vi "SunplusDailyYY.vi"() -> ()   [LabVIEW 2012]
uses:
  <vilib>/addons/database/Auxilliary.llb/DB Tools Cursor Type.ctl
  <vilib>/Utility/NIReport.llb/NI_report.lvclass
  <vilib>/addons/database/Connection.llb/DB Tools Open Connec (Path).vi
  <vilib>/addons/database/Connection.llb/Conn Execute.vi
  <vilib>/addons/database/Recordset.llb/Rec Fetch Recordset Data (R).vi
  <vilib>/addons/database/Recordset.llb/Rec Destroy - Connection.vi
  <vilib>/addons/database/_DB Variant To Data/Database Variant To Data.xnode
  <vilib>/addons/database/NI_Database_API.lvlib
  <vilib>/Utility/NIReport.llb/Excel/NI_Excel.lvclass
  <vilib>/Utility/SMTP/NI_SMTPEmail.lvlib
panel:
  out "error out 2":errorcluster
  in  "MIME content-type (application/octet-stream)":string="application/octet-stream"
  out "error out 4":errorcluster
  in  "?":cluster{"start row":i32, "start column":i32}
  out "error out":errorcluster
  in  "start (0, 0)":cluster{"start row":i32, "start column":i32}
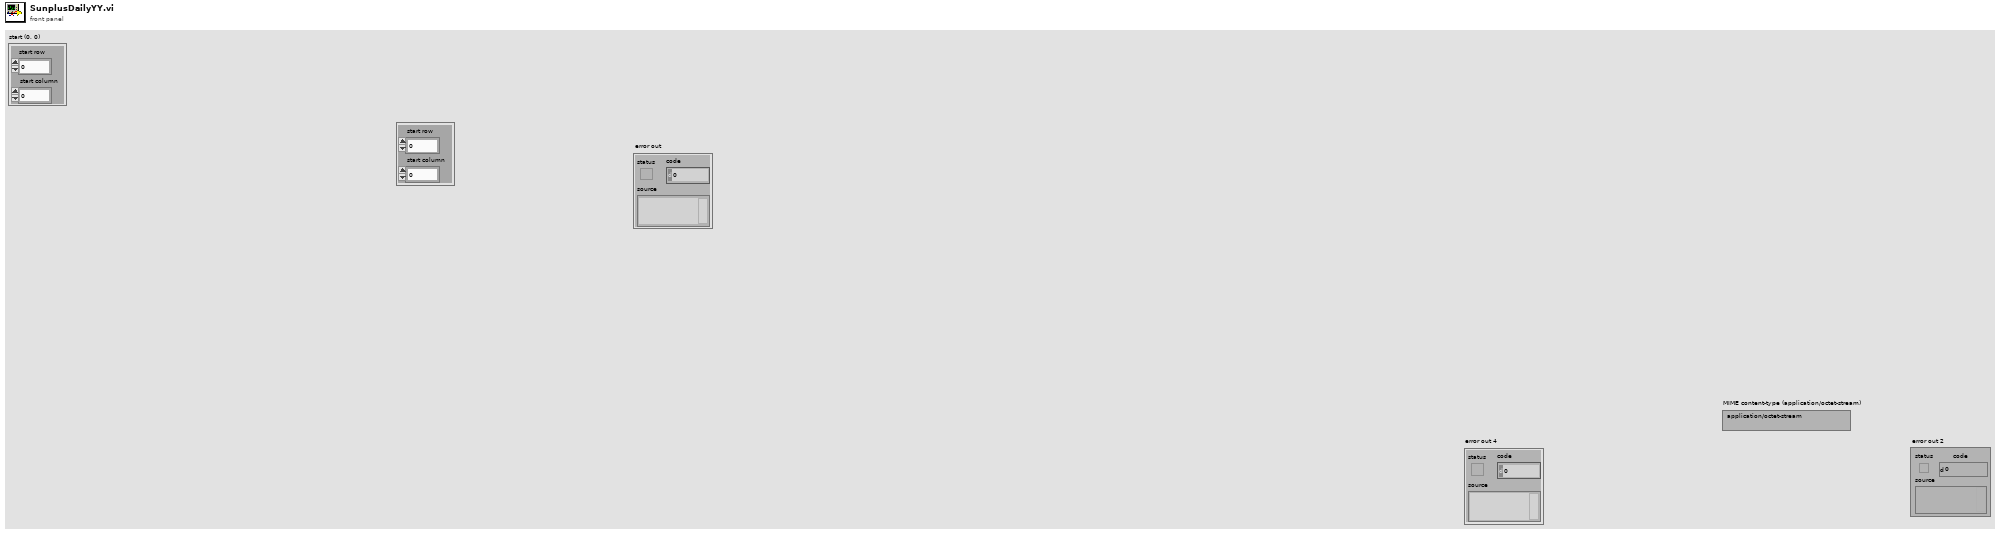
[diagram p1: front panel]
types:
  T1 = typedef "NI_Database_API.lvlib/DB Tools Cursor Type.ctl" = enum16{"forward-only", "keyset", "dynamic", "static"}
  T2 = enum16{"Standard Report", "HTML", "Word", "Excel"}
  T3 = typedef "NI_Database_API.lvlib/Conn ObjectReference.ctl" = refnum<k1>
  T4 = typedef "NI_Database_API.lvlib/Rec ObjectReference.ctl" = refnum<k1>
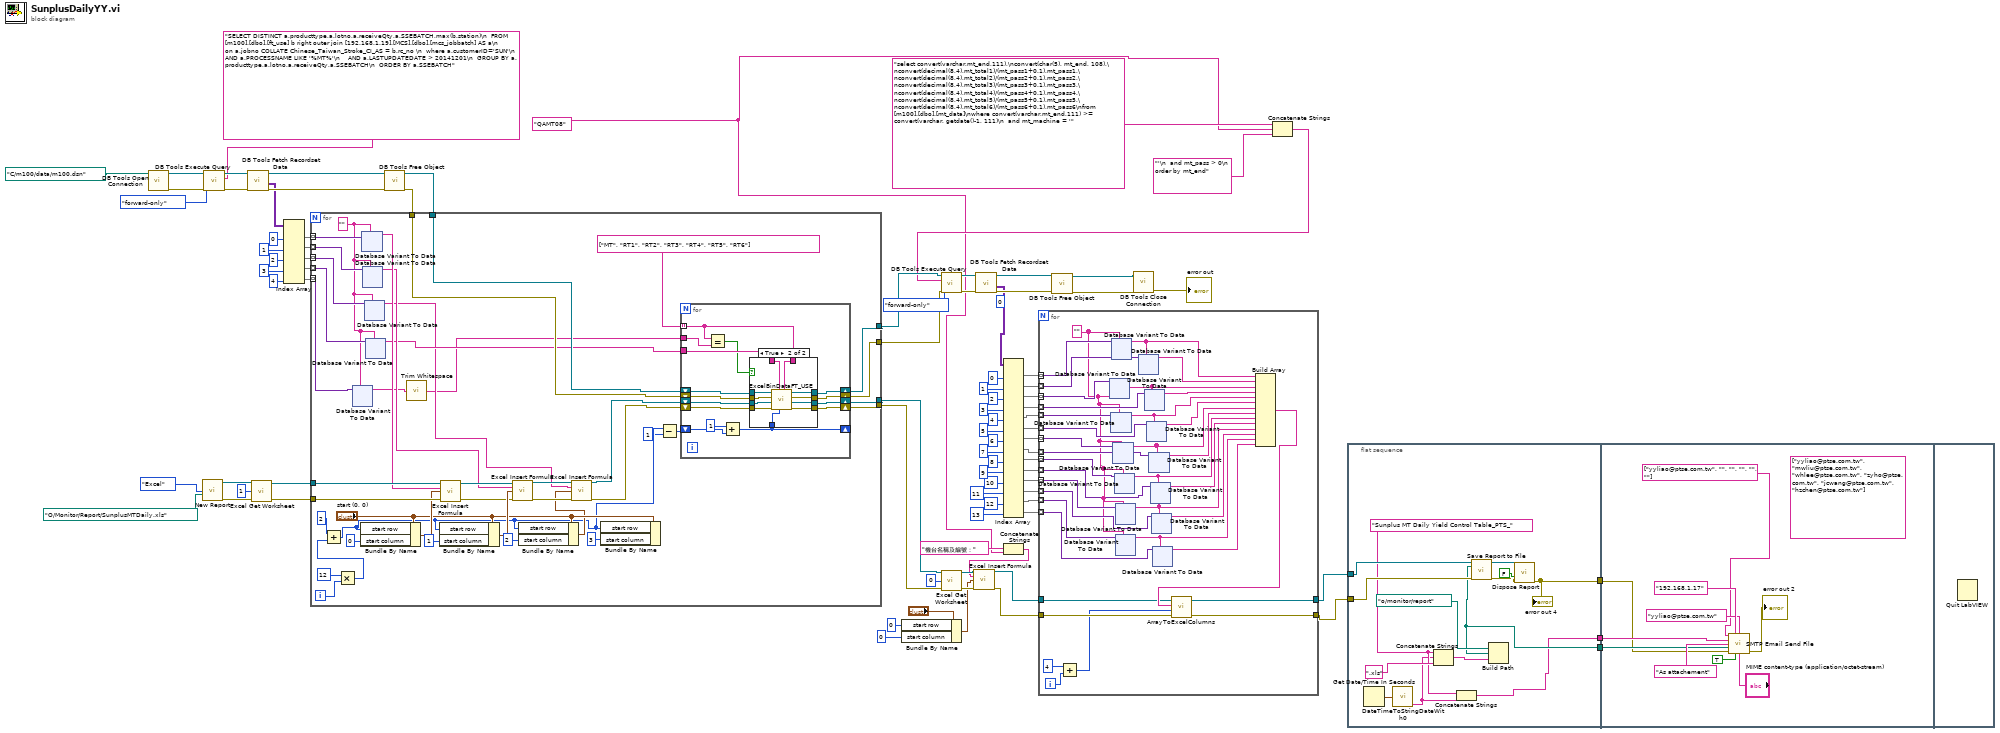
[diagram p0: block diagram]
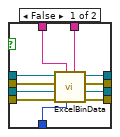
[diagram p2: hidden frame]
diagram:
  w6 = "QAMT08" ("Machine")
  (unwired) 0 ("index")
  n1 = call-poly <vilib>:"DB Tools Open Connection.vi"("connection information"=path "C:/m100/data/m100.dsn") -> ("error out"=w82:errorcluster, "connection reference"=w83:T3)  [unwired: 7 in]
  n2 = call <vilib>:"New Report.vi"("report type"=T2."Excel" ("Report Type"), "template (empty)"=path "O:/Monitor/Report/SunplusMTDaily.xls") -> ("report out"=w67:refnum<class "NI_report.lvclass">, "error out"=w66:errorcluster)  [unwired: 12 in]
  n3 = call-poly <vilib>:"DB Tools Execute Query.vi"("error in (no error)"=w82, "cursor type"=DB_Tools_Cursor_Type."forward-only", "SQL query"="SELECT DISTINCT a.producttype,a.lotno,a.receiveQty,a.SSEBATCH,max(b.station)\n  FROM [m100].[dbo].[ft_use] b right outer join [192.168.1.19].[MCS].[dbo].[mcs_jobbatch] AS a\n  on a.jobno COLLATE Chinese_Taiwan_Stroke_CI_AS = b.rc_no \n  where a.customerID='SUN'\n    AND a.PROCESSNAME LIKE '%MT%'\n    AND a.LASTUPDATEDATE > 20141201\n  GROUP BY a.producttype,a.lotno,a.receiveQty,a.SSEBATCH\n  ORDER BY a.SSEBATCH", "connection reference"=w83) -> ("error out"=w84:errorcluster, "recordset reference"=w85:T4)  [unwired: 4 in]
  n4 = call-poly <vilib>:"DB Tools Fetch Recordset Data.vi"("error in (no error)"=w84, "recordset reference"=w85) -> ("error out"=w86:errorcluster, "recordset data"=w79:variant[][], "recordset reference out"=w87:T4)  [unwired: 3 in]
  n5 = call <vilib>:"Excel Get Worksheet.vi"("report in"=w67, "worksheet index (0)"=1, "error in (no error)"=w66) -> ("report out"=w63:refnum<class "NI_report.lvclass">, "error out"=w62:errorcluster)  [unwired: 11 in]
  n6 = Index Array(array=w79, index (col) #1=0 ("disabled index (col)"), index (col) #2=1 ("index (col)"), index (col) #3=2 ("index (col)"), index (col) #4=3 ("index (col)"), index (col) #5=4 ("index (col)")) -> (element #1=w75:variant[], element #2=w74:variant[], element #3=w73:variant[], element #4=w69:variant[], element #5=w1:variant[])  [unwired: 5 in]
  n7 = call-poly <vilib>:"DB Tools Free Object.vi"("error in (no error)"=w86, "recordset reference"=w87) -> ("error out"=w72:errorcluster, "connection reference"=w71:T3)  [unwired: 8 in]
  n8 = for {
    tunnel: w75 -> [w132] mode=indexing
    tunnel: w74 -> [w131] mode=indexing
    tunnel: w73 -> [w130] mode=indexing
    tunnel: w72 -> [w107]
    tunnel: w71 -> [w108]
    tunnel: w69 -> [w129] mode=indexing
    tunnel: w63 -> [w128]
    tunnel: w62 -> [w127]
    tunnel: [w98] -> w61
    tunnel: [w97] -> w60
    tunnel: [w100] -> w52
    tunnel: [w99] -> w51
    tunnel: w1 -> [w94] mode=indexing
    i -> [w111]
    w93 = ""
    n9 = Multiply(x=12, y=w111) -> (x*y=w109:i32)
    n10 = Add(x=2, y=w109) -> (x+y=w104:i32)
    n11 = xnode "Database Variant To Data"("database variant"=w94, "type"=w93) -> ("data"=w92:string)  [unwired: 1 in, 1 out]
    n12 = Bundle By Name(cluster="start (0, 0)", "start row"=w104, "start column"=0) -> (w126:cluster{"start row":i32, "start column":i32})
    n13 = xnode "Database Variant To Data"("database variant"=w132, "type"=w93) -> ("data"=w123:string)  [unwired: 1 in, 1 out]
    n14 = xnode "Database Variant To Data"("database variant"=w131, "type"=w93) -> ("data"=w118:string)  [unwired: 1 in, 1 out]
    n15 = xnode "Database Variant To Data"("database variant"=w130, "type"=w93) -> ("data"=w95:string)  [unwired: 1 in, 1 out]
    n16 = xnode "Database Variant To Data"("database variant"=w129, "type"=w93) -> ("data"=w101:string)  [unwired: 1 in, 1 out]
    n17 = call <vilib>:"Trim Whitespace.vi"("string"=w92) -> ("trimmed string"=w91:string)  [unwired: 1 in]
    n18 = Bundle By Name(cluster="start (0, 0)", "start row"=w104, "start column"=1) -> (w121:cluster{"start row":i32, "start column":i32})
    n19 = call <vilib>:"Excel Insert Formula.vi"("report in"=w128, "formula"=w123, "start (0, 0)"=w126, "error in (no error)"=w127) -> ("report out"=w120:refnum<class "NI_report.lvclass">, "error out"=w119:errorcluster)  [unwired: 10 in]
    n20 = call <vilib>:"Excel Insert Formula.vi"("report in"=w120, "formula"=w118, "start (0, 0)"=w121, "error in (no error)"=w119) -> ("report out"=w116:refnum<class "NI_report.lvclass">, "error out"=w115:errorcluster)  [unwired: 10 in]
    n21 = Bundle By Name(cluster="start (0, 0)", "start row"=w104, "start column"=2) -> (w112:cluster{"start row":i32, "start column":i32})
    n22 = call <vilib>:"Excel Insert Formula.vi"("report in"=w116, "formula"=w95, "start (0, 0)"=w112, "error in (no error)"=w115) -> ("report out"=w106:refnum<class "NI_report.lvclass">, "error out"=w105:errorcluster)  [unwired: 10 in]
    n23 = Bundle By Name(cluster="start (0, 0)", "start row"=w104, "start column"=3) -> ()  [unwired: 1 out]
    n24 = Subtract(x=w104, y=1) -> (x-y=w102:i32)
    n25 = for {
      shift-right: [w178] -> w100
      shift-left: w108 -> [w171]
      shift-right: [w177] -> w99
      shift-left: w107 -> [w170]
      shift-right: [w176] -> w98
      shift-left: w106 -> [w169]
      shift-right: [w175] -> w97
      shift-left: w105 -> [w168]
      shift-right: [w174] -> _
      shift-left: w102 -> [w173]
      tunnel: w101 -> [w172]
      tunnel: string[] ["MT", "RT1", "RT2", "RT3", "RT4", "RT5", "RT6"] ("Array") -> [w166] mode=indexing
      tunnel: w91 -> [w167]
      n26 = Equal?(x=w166, y=w167) -> (x = y?=w165:bool)
      n27 = Add(x=1, y=w173) -> (x+y=w174:i32)
      n28 = case shown="True" w165 {
        tunnel: [w190 w196] -> w178
        tunnel: [w189 w195] -> w177
        tunnel: [w188 w194] -> w176
        tunnel: [w187 w193] -> w175
        tunnel: w174 -> [w186 w201]
        tunnel: w172 -> [w185 w192]
        tunnel: w171 -> [w184 w200]
        tunnel: w170 -> [w183 w199]
        tunnel: w169 -> [w182 w198]
        tunnel: w168 -> [w181 w197]
        tunnel: w166 -> [w180 w191]
        frame False {
          n29 = call "ExcelBinData.vi"("step"=w180, "start row"=w186, "jobno"=w185, "error in (no error) 2"=w181, "report in"=w182, "error in (no error)"=w183, "connection reference 2"=w184) -> ("error out 2"=w187:errorcluster, "report out"=w188:refnum<class "NI_report.lvclass">, "error out"=w189:errorcluster, "connection reference"=w190:T3)  [unwired: 1 in]
        }
        frame True {
          n30 = call "ExcelBinDataFT_USE.vi"("step"=w191, "start row"=w201, "jobno"=w192, "error in (no error) 2"=w197, "report in"=w198, "error in (no error)"=w199, "connection reference 2"=w200) -> ("error out 2"=w193:errorcluster, "report out"=w194:refnum<class "NI_report.lvclass">, "error out"=w195:errorcluster, "connection reference"=w196:T3)  [unwired: 1 in]
        }
      }
    }
  }
  n31 = Bundle By Name(cluster="?", "start row"=0, "start column"=0) -> (w11:cluster{"start row":i32, "start column":i32})
  n32 = call <vilib>:"Excel Get Worksheet.vi"("report in"=w61, "worksheet index (0)"=0, "error in (no error)"=w60) -> ("report out"=w16:refnum<class "NI_report.lvclass">, "error out"=w15:errorcluster)  [unwired: 11 in]
  n33 = Concatenate Strings("機台名稱及編號：" ("formula"), w6) -> (w8:string)
  n34 = call <vilib>:"Excel Insert Formula.vi"("report in"=w16, "formula"=w8, "start (0, 0)"=w11, "error in (no error)"=w15) -> ("report out"=w10:refnum<class "NI_report.lvclass">, "error out"=w9:errorcluster)  [unwired: 10 in]
  n35 = Concatenate Strings("select convert(varchar,mt_end,111),\nconvert(char(5), mt_end, 108),\nconvert(decimal(8,4),mt_total1)/(mt_pass1+0.1),mt_pass1,\nconvert(decimal(8,4),mt_total2)/(mt_pass2+0.1),mt_pass2,\nconvert(decimal(8,4),mt_total3)/(mt_pass3+0.1),mt_pass3,\nconvert(decimal(8,4),mt_total4)/(mt_pass4+0.1),mt_pass4,\nconvert(decimal(8,4),mt_total5)/(mt_pass5+0.1),mt_pass5,\nconvert(decimal(8,4),mt_total6)/(mt_pass6+0.1),mt_pass6\nfrom [m100].[dbo].[mt_data]\nwhere convert(varchar,mt_end,111) >= convert(varchar, getdate()-1, 111)\n  and mt_machine = '" ("SQL query"), w6, "'\n  and mt_pass > 0\n  order by mt_end" ("SQL query")) -> (w17:string)
  n36 = call-poly <vilib>:"DB Tools Execute Query.vi"("error in (no error)"=w51, "cursor type"=DB_Tools_Cursor_Type."forward-only", "SQL query"=w17, "connection reference"=w52) -> ("error out"=w58:errorcluster, "recordset reference"=w57:T4)  [unwired: 4 in]
  n37 = call-poly <vilib>:"DB Tools Fetch Recordset Data.vi"("error in (no error)"=w58, "recordset reference"=w57) -> ("error out"=w55:errorcluster, "recordset data"=w48:variant[][], "recordset reference out"=w56:T4)  [unwired: 3 in]
  n38 = Index Array(array=w48, index (col) #1=0 ("disabled index (col)"), index (col) #2=1 ("index (col)"), index (col) #3=2 ("index (col)"), index (col) #4=3 ("index (col)"), index (col) #5=4 ("index (col)"), index (col) #6=5 ("index (col)"), index (col) #7=6 ("index (col)"), index (col) #8=7 ("index (col)"), index (col) #9=8 ("index (col)"), index (col) #10=9 ("index (col)"), index (col) #11=10 ("index (col)"), index (col) #12=11 ("index (col)"), index (col) #13=12 ("index (col)"), index (col) #14=13 ("index (col)")) -> (element #1=w45:variant[], element #2=w44:variant[], element #3=w43:variant[], element #4=w32:variant[], element #5=w31:variant[], element #6=w30:variant[], element #7=w29:variant[], element #8=w28:variant[], element #9=w27:variant[], element #10=w26:variant[], element #11=w25:variant[], element #12=w24:variant[], element #13=w21:variant[], element #14=w20:variant[])  [unwired: 14 in]
  n39 = for {
    tunnel: w45 -> [w366] mode=indexing
    tunnel: w44 -> [w365] mode=indexing
    tunnel: w43 -> [w364] mode=indexing
    tunnel: w32 -> [w362] mode=indexing
    tunnel: w31 -> [w358] mode=indexing
    tunnel: w30 -> [w356] mode=indexing
    tunnel: w29 -> [w354] mode=indexing
    tunnel: w28 -> [w351] mode=indexing
    tunnel: w27 -> [w350] mode=indexing
    tunnel: w26 -> [w349] mode=indexing
    tunnel: w25 -> [w346] mode=indexing
    tunnel: w24 -> [w345] mode=indexing
    tunnel: w21 -> [w342] mode=indexing
    tunnel: w20 -> [w341] mode=indexing
    tunnel: w10 -> [w336]
    tunnel: w9 -> [w335]
    tunnel: [w331] -> w5
    tunnel: [w330] -> w4
    i -> [w334]
    w338 = ""
    n40 = Add(x=4, y=w334) -> (x+y=w332:i32)
    n41 = xnode "Database Variant To Data"("database variant"=w364, "type"=w338) -> ("data"=w360:string)  [unwired: 1 in, 1 out]
    n42 = xnode "Database Variant To Data"("database variant"=w358, "type"=w338) -> ("data"=w357:string)  [unwired: 1 in, 1 out]
    n43 = xnode "Database Variant To Data"("database variant"=w366, "type"=w338) -> ("data"=w361:string)  [unwired: 1 in, 1 out]
    n44 = xnode "Database Variant To Data"("database variant"=w354, "type"=w338) -> ("data"=w353:string)  [unwired: 1 in, 1 out]
    n45 = xnode "Database Variant To Data"("database variant"=w350, "type"=w338) -> ("data"=w348:string)  [unwired: 1 in, 1 out]
    n46 = xnode "Database Variant To Data"("database variant"=w346, "type"=w338) -> ("data"=w344:string)  [unwired: 1 in, 1 out]
    n47 = xnode "Database Variant To Data"("database variant"=w342, "type"=w338) -> ("data"=w340:string)  [unwired: 1 in, 1 out]
    n48 = xnode "Database Variant To Data"("database variant"=w365, "type"=w361) -> ("data"=w363:string)  [unwired: 1 in, 1 out]
    n49 = xnode "Database Variant To Data"("database variant"=w362, "type"=w360) -> ("data"=w359:string)  [unwired: 1 in, 1 out]
    n50 = xnode "Database Variant To Data"("database variant"=w356, "type"=w357) -> ("data"=w355:string)  [unwired: 1 in, 1 out]
    n51 = xnode "Database Variant To Data"("database variant"=w351, "type"=w353) -> ("data"=w352:string)  [unwired: 1 in, 1 out]
    n52 = xnode "Database Variant To Data"("database variant"=w349, "type"=w348) -> ("data"=w347:string)  [unwired: 1 in, 1 out]
    n53 = xnode "Database Variant To Data"("database variant"=w345, "type"=w344) -> ("data"=w343:string)  [unwired: 1 in, 1 out]
    n54 = xnode "Database Variant To Data"("database variant"=w341, "type"=w340) -> ("data"=w339:string)  [unwired: 1 in, 1 out]
    n55 = Build Array(w361, w363, w360, w359, w357, w355, w353, w352, w348, w347, w344, w343, w340, w339) -> (w337:string[])
    n56 = call "ArrayToExcelColumns.vi"("error in (no error)"=w335, "start row"=w332, "ArrayData"=w337, "report in"=w336) -> ("error in (no error) 2"=w330:errorcluster, "report in 2"=w331:refnum<class "NI_report.lvclass">)  [unwired: 6 in]
  }
  n57 = call-poly <vilib>:"DB Tools Free Object.vi"("error in (no error)"=w55, "recordset reference"=w56) -> ("error out"=w53:errorcluster, "connection reference"=w54:T3)  [unwired: 8 in]
  n58 = call <vilib>:"DB Tools Close Connection.vi"("error in (no error)"=w53, "connection reference"=w54) -> ("error out"=→"error out":errorcluster)  [unwired: 5 in]
  n59 = flat-sequence {
    tunnel: w5 -> [w824]
    tunnel: w4 -> [w823]
    tunnel: [w815] -> w90
    tunnel: [w819] -> w89
    tunnel: [w818] -> w88
    tunnel: w90 -> [w832]
    tunnel: w89 -> [w831]
    tunnel: w88 -> [w830]
    frame #0 {
      w817 = "Sunplus MT Daily Yield Control Table_PTS_" ("string")
      n60 = Get Date/Time In Seconds() -> (seconds since 1Jan1904=w821:timestamp)
      n61 = call "DateTimeToStringDateWith0.vi"("time stamp"=w821) -> ("Dateyyyymmdd"=w816:string)  [unwired: 9 in, 1 out]
      n62 = Concatenate Strings(w817, w816, ".xls" ("string")) -> (w820:string)
      n63 = Concatenate Strings(w817, w816) -> (w815:string)
      n64 = Build Path(base path=path "o:/monitor/report", name or relative path=w820) -> (appended path=w819:path)
      n65 = call-dynamic "Save Report to File.vi"("report in"=w824, "report file path"=w819, "error in (no error)"=w823) -> ("report out"=w826:refnum<class "NI_report.lvclass">, "error out"=w825:errorcluster)  [unwired: 11 in]
      n66 = call-dynamic "Dispose Report.vi"("report in"=w826, "save changes? (F)"=FALSE, "error in (no error)"=w825) -> ("error out"=w818:errorcluster)  [unwired: 12 in]
      "error out 4" <- w818
    }
    frame #1 {
      (unwired) string[] ["yyliao@ptse.com.tw", "mwliu@ptse.com.tw", "whlee@ptse.com.tw", "zyho@ptse.com.tw", "jcwang@ptse.com.tw", "hzchen@ptse.com.tw"] ("recipients")
      n67 = call <vilib>:"SMTP Email Send File.vi"("recipients"=string[] ["yyliao@ptse.com.tw", "", "", "", "", ""], "mail server"="192.168.1.17", "return address"="yyliao@ptse.com.tw", "subject ([No Subject])"=w832, "message"="As attachement", "file path"=w831, "error in (no error)"=w830, "binary? (F)"=TRUE, "MIME content-type (application/octet-stream)"="MIME content-type (application/octet-stream)") -> ("error out"=→"error out 2":errorcluster)  [unwired: 5 in, 1 out]
    }
    frame #2 {
      n68 = Quit LabVIEW() -> ()  [unwired: 1 in]
    }
  }
